vi "Run.vi"(8 "error in (no error)":errorcluster caption="entrée d'erreur (pas d'erreur)", 9 "labels_pred":string[][](array[string]), 10 "labels_true":string[][](array[string]), 11 "Adjusted_Mutual_Info_Score.lvclass":refnum<class "Adjusted_Mutual_Info_Score.lvclass">) -> (0 "error out":errorcluster caption="sortie d'erreur", 2 "String Data":string, 3 "Adjusted_Mutual_Info_Score.lvclass":refnum<class "Adjusted_Mutual_Info_Score.lvclass">)   [LabVIEW 2020, in "Adjusted_Mutual_Info_Score.lvclass"]
doc: "Returns :\n\n- ami : float (upperlimited by 1.0)\nThe AMI returns a value of 1 when the two partitions are identical (ie perfectly matched). Random partitions (independent labellings) have an expected AMI around 0 on average hence can be negative."
uses:
  Adjusted_Mutual_Info_Score.lvclass
  Adjusted_Mutual_Info_Score.lvclass/Adjusted_Mutual_Info_Score.ctl
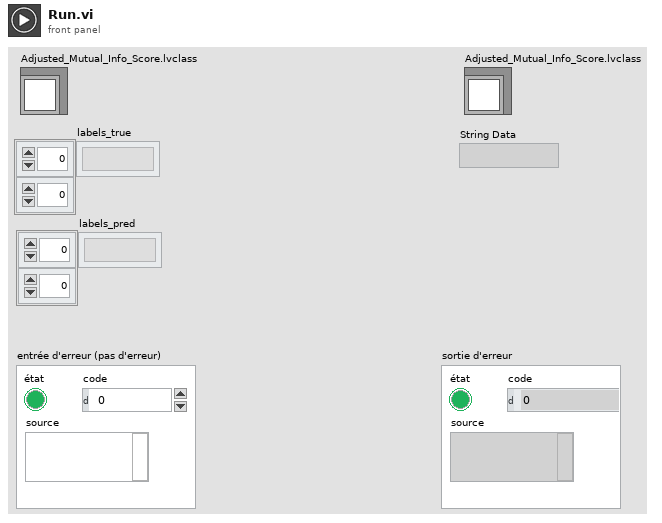
[diagram p1: front panel]
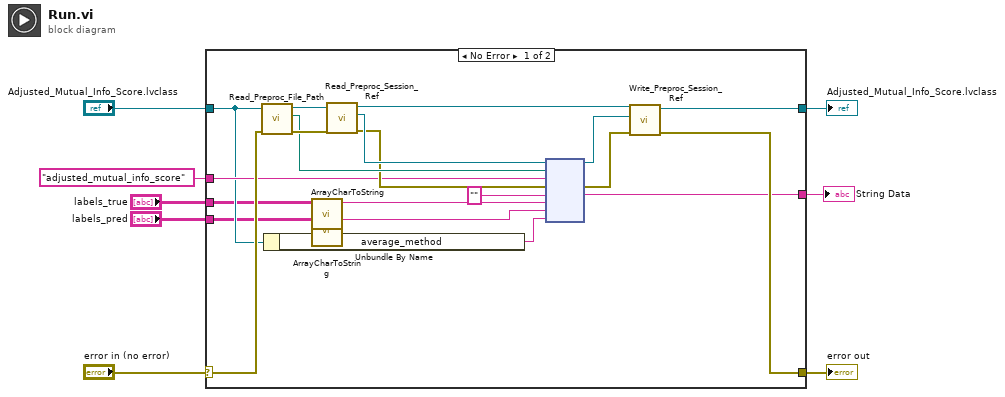
[diagram p0: block diagram]
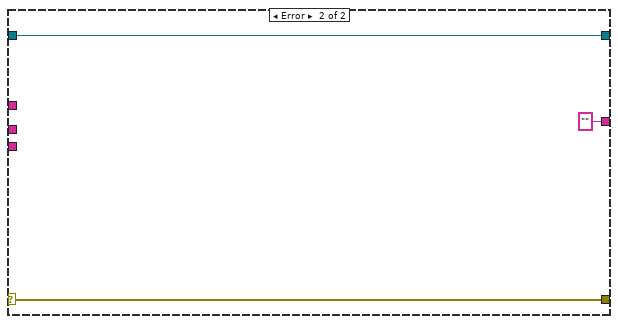
[diagram p2: hidden frame]
diagram:
  n1 = case shown="No Error" "error in (no error)" {
    selector: "error in (no error)" -> [w18 w31]
    tunnel: [w19 w31] -> w7
    tunnel: [w13 w30] -> w5
    tunnel: "Adjusted_Mutual_Info_Score.lvclass" -> [w16 w30]
    tunnel: "adjusted_mutual_info_score" -> [w17 _]
    tunnel: [w14 ""] -> w4
    tunnel: "labels_true" -> [w12 _]
    tunnel: "labels_pred" -> [w10 _]
    frame No Error {
      n2 = call-dynamic "Read_Preproc_File_Path.vi"("error in (no error)"=w18, "Python in"=w16) -> ("error out"=w27:errorcluster, "File_Path"=w26:path, "Python out"=w28:refnum<class "Adjusted_Mutual_Info_Score.lvclass">)  [unwired: 7 in]
      n3 = Unbundle By Name(w16) -> ("average_method"=w15:string)
      n4 = call "ArrayCharToString.vi"("TAB"=w12) -> ("Instruction"=w11:string)  [unwired: 10 in]
      n5 = call "ArrayCharToString.vi"("TAB"=w10) -> ("Instruction"=w9:string)  [unwired: 10 in]
      n6 = call-dynamic "Read_Preproc_Session_Ref.vi"("error in (no error)"=w27, "Python in"=w28) -> ("error out"=w24:errorcluster, "Session_ref"=w25:refnum<k35>, "Python out"=w23:refnum<class "Adjusted_Mutual_Info_Score.lvclass">)  [unwired: 7 in]
      n7 = node(w25, w26, w17, w24, "", w11, w9, w15) -> (w21:refnum<k35>, w22:errorcluster, w14:string)  [unwired: 3 in, 2 out]
      n8 = call-dynamic "Write_Preproc_Session_Ref.vi"("error in (no error)"=w22, "Session_ref"=w21, "Python in"=w23) -> ("error out"=w19:errorcluster, "Python out"=w13:refnum<class "Adjusted_Mutual_Info_Score.lvclass">)  [unwired: 7 in]
    }
    frame Error {
    }
  }
  "error out" <- w7
  "Adjusted_Mutual_Info_Score.lvclass" <- w5
  "String Data" <- w4
